vi "Get VI Path from Tree.vi"(10 "Tree Selection":string, 11 "Tree Map":T1) -> (2 "path":path, 3 "found?":bool)   [LabVIEW 2020, in "Panther Dashboard.lvlib"]
uses:
  Panther Dashboard.lvlib
  <vilib>/National Instruments/Tree Map/Tree Map Data.ctl
  <vilib>/National Instruments/Tree Map/Tree Map.lvlib
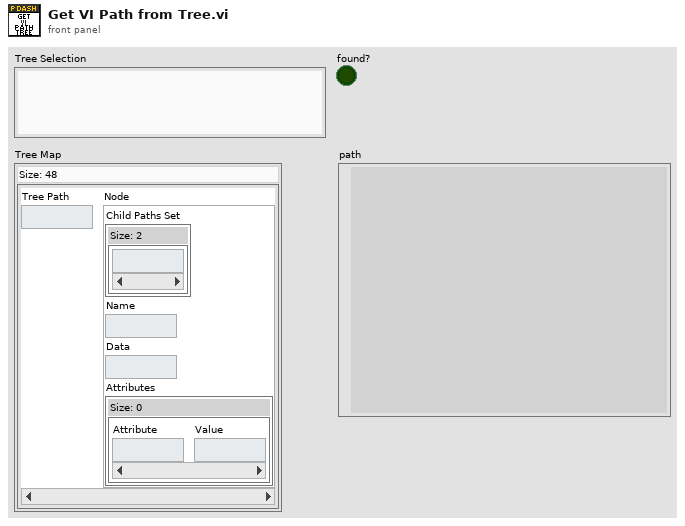
[diagram p1: front panel]
types:
  T1 = typedef "Tree Map.lvlib/Tree Map Data.ctl" = map{string, cluster{"Child Paths Set":set{string}, "Name":string, "Data":string, "Attributes":map{string, string}}}
  T2 = cluster{"Child Paths Set":set{string}, "Name":string, "Data":string, "Attributes":map{string, string}}
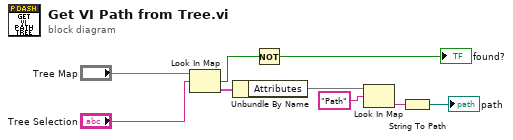
[diagram p0: block diagram]
diagram:
  n1 = Look In Map(map="Tree Map", key="Tree Selection") -> (key not found?=w6:bool, value=w7:T2)  [unwired: 1 in]
  n2 = Unbundle By Name(w7) -> ("Attributes"=w5:map{string, string})
  n3 = Not(x=w6) -> (.not. x?=→"found?":bool)
  n4 = Look In Map(map=w5, key="Path") -> (value=w3:string)  [unwired: 1 in, 1 out]
  n5 = String To Path(string=w3) -> (path=→"path":path)
